vi "Cal Pos Passed.vi"(8 "error in (no error)":errorcluster, 9 "Init-Enc-Pos(cnt)":dbl, 10 "Current-Enc-Pos(cnt)":dbl, 11 "Enc-Coefficient":dbl) -> (0 "error out":errorcluster, 3 "Pos Passed(deg)":dbl)   [LabVIEW 2013, in "SGDV_Ctrl_v13_lib.lvlib"]
uses:
  SGDV_Ctrl_v13_lib.lvlib
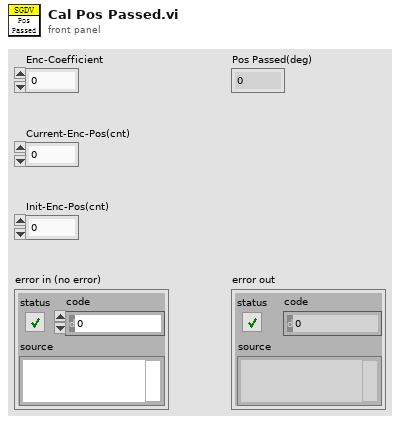
[diagram p1: front panel]
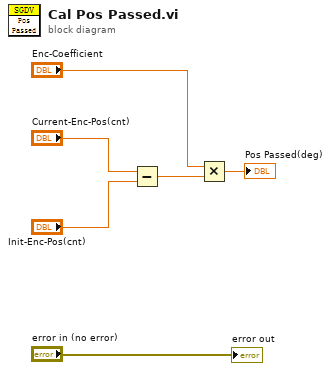
[diagram p0: block diagram]
diagram:
  n1 = Subtract(x="Current-Enc-Pos(cnt)", y="Init-Enc-Pos(cnt)") -> (x-y=w3:dbl)
  n2 = Multiply(x="Enc-Coefficient", y=w3) -> (x*y=→"Pos Passed(deg)":dbl)
  "error out" <- "error in (no error)"
